vi "checkDeadband.vi"(1 "tolerance":dbl, 2 "input":dbl) -> (6 "output":bool)   [LabVIEW 2011]
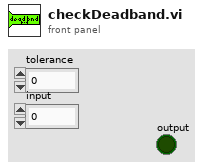
[diagram p1: front panel]
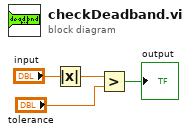
[diagram p0: block diagram]
diagram:
  n1 = Absolute Value(x="input") -> (abs(x)=w3:dbl)
  n2 = Greater?(x=w3, y="tolerance") -> (0:→"output":bool)
